vi "Cluster to VArray.vi"(8 "error in (no error)":errorcluster, 10 "Cluster":refnum<class "variant.lvclass">) -> (0 "error out":errorcluster, 2 "VArray":refnum<class "variant.lvclass">)   [LabVIEW 2020, in "variant.lvlib" / "variant.lvclass"]
doc: "Convert a cluster of identical element datatypes into an array."
uses:
  variant.lvclass
  variant.lvclass/variant.ctl
  Type Descriptor/TD.lvclass/TD.ctl
  Bytes/Bytes.lvclass/Bytes.ctl
  Type Descriptor Enumeration.ctl
  Type Descriptor/TD.lvclass
  C:/projects/OpenG-Variant-Data-Library/source/library/Bytes/Bytes.lvclass
  5d20640f-5bd6-45d0-abcc-d5dfbfc7c14e.vi
  Bytes/to_data.vi
  Type Descriptor/get_num_elements.vi/b3898c1b-5169-4cb1-894b-457c92b4a1c3.vi
  Bytes/from_byte_array.vi
  Type Descriptor/get_num_elements.vi/b3898c1b-5169-4cb1-894b-457c92b4a1c3.vi/81433c74-ee36-47cf-a886-10c868675b30.vi
  Type Descriptor/get_num_elements.vi/b3898c1b-5169-4cb1-894b-457c92b4a1c3.vi/d8d9ff34-2c15-4edb-a5ad-7260f11560db.vi
  DataString/DataString.lvclass
  Bytes/Bytes.lvclass
  <userlib>/_OpenG.lib/error/error.llb/openg_error.lvlib
  openg_variant.lvlib
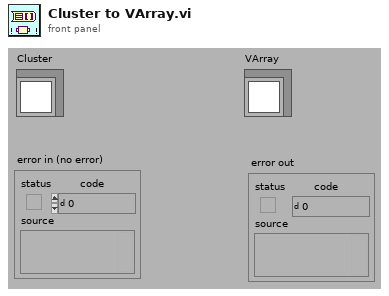
[diagram p1: front panel]
types:
  T1 = typedef "openg_variant.lvlib/Type Descriptor Enumeration.ctl" = enum8{"<Null>", "I8", "I16", "I32", "I64", "U8", "U16", "U32", "U64", "SGL", "DBL", "EXT", "CSG", "CDB", "CXT", "0x0F", "0x10", "0x11", "0x12", "0x13", "0x14", "Enum U8", "Enum U16", "Enum U32", "Enum U64", "SGL PQ", "DBL PQ", "EXT PQ", "CSG PQ", "CDB PQ", "CXT PQ", "0x1F", "0x20", "Boolean", "0x22", "0x23", "0x24", "0x25", "0x26", "0x27", "0x28", "0x29", "0x2A", "0x2B", "0x2C", "0x2D", "0x2E", "0x2F", "String", "0x31", "Path", "Pict", "0x34", "0x35", "0x36", "DAQ", "0x38", "0x39", "0x3A", "0x3B", "0x3C", "0x3D", "0x3E", "0x3F", "Array", "0x41", "0x42", "0x43", "0x44", "0x45", "0x46", "0x47", "0x48", "0x49", "0x4A", "0x4B", "0x4C", "0x4D", "0x4E", "0x4F", "Cluster", "0x51", "0x52", "Variant", "Waveform", "0x55", "0x56", "0x57", "0x58", "0x59", "0x5A", "0x5B", "0x5C", "0x5D", "0x5E", "Fixed Point", "0x60", "0x61", "0x62", "0x63", "0x64", "0x65", "0x66", "0x67", "0x68", "0x69", "0x6A", "0x6B", "0x6C", "0x6D", "0x6E", "0x6F", "Refnum", "0x71", "0x72", "Set Collection", "Map Collection"}
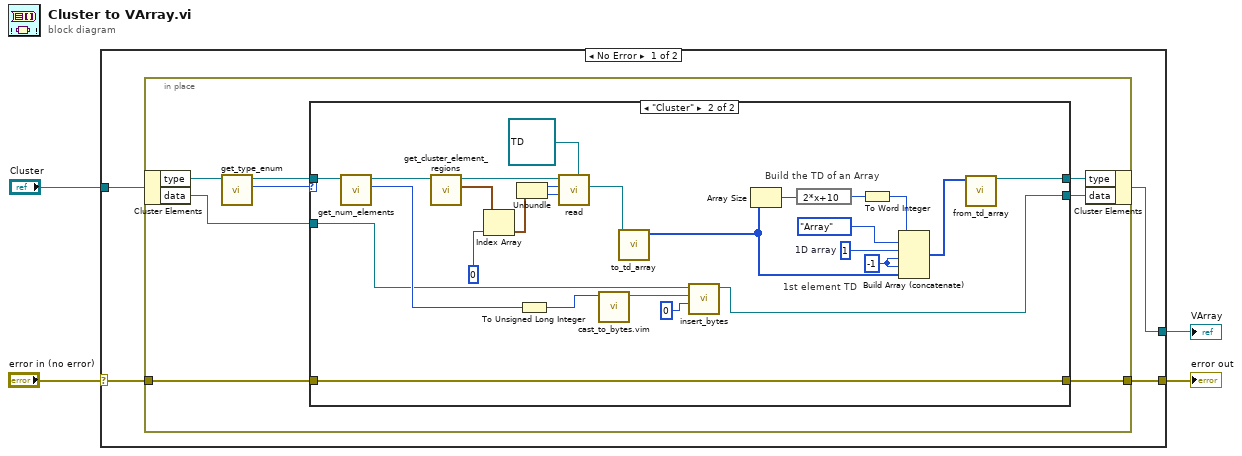
[diagram p0: block diagram]
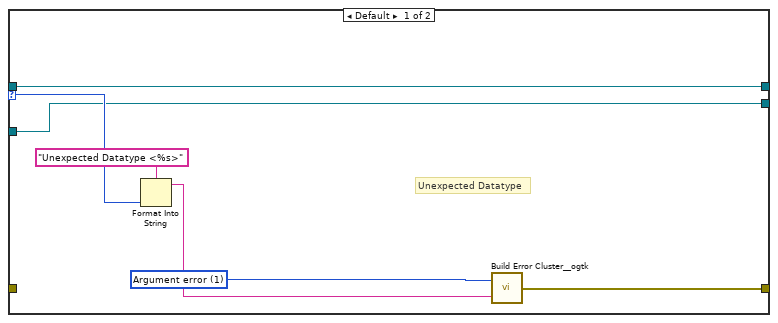
[diagram p2: hidden frame]
diagram:
  n1 = case shown="No Error" "error in (no error)" {
    selector: "error in (no error)" -> [w5 w50]
    tunnel: [w8 w50] -> w4
    tunnel: [w6 _] -> w2
    tunnel: "Cluster" -> [w7 _]
    frame No Error {
      n2 = in-place {
        in-place-border: [w16] -> w8
        in-place-border: w5 -> [w9]
        n3 = in-place-cluster #1(w7) -> ("type"=w15:refnum<class "TD.lvclass">, "data"=w12:refnum<class "DataString.lvclass">)
        n4 = call "get_type_enum.vi"("TypeDescriptor"=w15) -> ("type"=w14:T1, "TypeDescriptor out"=w13:refnum<class "TD.lvclass">)  [unwired: 9 in]
        n5 = case shown="\"Cluster\"" w14 {
          selector: w14 -> [w20 _]
          tunnel: [w23 w24] -> w16
          tunnel: w13 -> [w18 w43]
          tunnel: w12 -> [w17 w31]
          tunnel: [w18 w26] -> w11
          tunnel: [w17 w25] -> w10
          tunnel: w9 -> [_ w24]
          frame Default {
            w22 = 1 items=["No error", "Argument error", "Memory is full", "Out of zone", "End of file", "File already open", "Generic file I/O error", "File not found", "File permission error", "Disk is full", "Duplicate path", "Too many files open", "System feature not enabled", "Resource file not found", "Cannot add resource", "Resource not found", "Image not found", "Image memory error", "Pen does not exist", "Config type invalid", "Config token not found", "Config parse error", "Config memory error", "Bad external code format", "Bad external code offset", "External code not present", "Null window", "Destroy window error", "Null menu", "Print aborted", "Bad print record", "Print driver error", "Windows error during printing", "Memory error during printing", "Print dialog error", "Generic print error", "Invalid device refnum", "Device not found", "Device parameter error", "Device unit error", "Cannot open device", "Device call aborted", "Generic error", "Cancelled by user", "Object ID too low", "Object ID too high", "Object not in heap", "Unknown heap", "Unknown object (invalid DefProc)", "Unknown object (DefProc not in table)", "Message out of range", "Invalid (null) method", "Unknown message", "Manager call not supported", "Bad address", "Network operation in progress", "Network operation timed out", "Connection is busy", "Network attribute not supported", "Network error", "Address in use", "System out of memory", "Connection aborted", "Connection refused", "Not connected", "Already connected", "Connection closed", "Initialization error (interapplication manager)", "Bad occurrence", "Wait on unbound occurrence handler", "Occurrence queue overflow", "Datalog type conflict", "Unused", "Unrecognized type (interapplication manager)", "Memory corrupt", "Failed to make temporary DLL", "Old CIN version", "Drag socket not found", "Failed to load drop-object", "Failed to register OLE object", "Failed to release OLE object", "Format specifier type mismatch", "Unknown format specifier", "Too few format specifiers", "Too many format specifiers", "Scan failed", "Newer CIN version", "Error converting to variant", "Runtime menu error", "Password tampered", "Variant attribute not found", "Incompatible variant data type", "Event data is not available", "Event Store is not present", "Occurrence is not found", "Event Queue is not created", "Event info is not available", "Refnum passed is NULL", "Error retrieving Class GUID", "Error retrieving CoClass GUID", "Error retrieving TypeLib GUID.", "Bad built application magic bytes.", "Specific driver is different from the specific driver associated with the Logical Name.", "There is no session opened to the class driver.", "Max Error", "MAX - Error with config objects", "MAX - Error loading configuration", "MAX - Group not supported"]
            # "Unexpected Datatype"
            n6 = Format Into String(format string="Unexpected Datatype <%s>" ("Format String"), w20) -> (resulting string=w19:string)  [unwired: 2 in, 1 out]
            n7 = call <userlib>:"Build Error Cluster__ogtk.vi"("String to Prepend to source (\"\")"=w19, "code"=w22) -> ("error out"=w23:errorcluster)
          }
          frame "Cluster" {
            w47 = i16 -1 ("Input Element")
            w48 = i16 1  # 1D array
            # "Build the TD of an Array"
            # "1st element TD"
            n8 = call "get_num_elements.vi"("TypeDescriptor"=w43) -> ("num_element"=w42:i32, "TypeDescriptor out"=w41:refnum<class "TD.lvclass">)  [unwired: 9 in]
            n9 = call "get_cluster_element_regions.vi"("TypeDescriptor"=w41) -> ("element_regions"=w40:cluster{i32, i32}[], "TypeDescriptor out"=w39:refnum<class "TD.lvclass">)  [unwired: 8 in, 1 out]
            n10 = Index Array(array=w40, index=0 ("Index")) -> (element=w37:cluster{i32, i32})
            n11 = Unbundle(w37) -> (w35:i32, w36:i32)
            n12 = To Unsigned Long Integer(number=w42) -> (unsigned 32bit integer=w30:u32)
            n13 = call "read.vi"("type to read"=refnum<class "TD.lvclass"> refnum ("TypeDescriptor in"), "length (-1: rest)"=w36, "offset (-1: current position)"=w35, "Bytes in"=w39) -> ("Bytes read"=w34:refnum<class "TD.lvclass">)  [unwired: 6 in, 1 out]
            n14 = call "cast_to_bytes.vim"("anything"=w30) -> ("bytes"=w29:refnum<class "Bytes.lvclass">)  [unwired: 10 in]
            n15 = call "to_td_array.vi"("TypeDescriptor in"=w34) -> ("type string"=w32:i16[])  [unwired: 10 in]
            n16 = call "insert_bytes.vi"("offset (-1: current position)"=0, "bytes to insert"=w29, "Bytes in"=w31) -> ("Bytes out"=w25:refnum<class "DataString.lvclass">)  [unwired: 8 in]
            n17 = Array Size(array=w32) -> (size(s)=w46:i32)
            n18 = expression code="2*x+10"(w46) -> (w45:i32)
            n19 = To Word Integer(number=w45) -> (16bit integer=w44:i16)
            n20 = Build Array (concatenate)(w44, Type_Descriptor_Enumeration."Array" ("Type Descriptor Enumeration"), w48, w47, w47, w32) -> (w27:i16[])
            n21 = call "from_td_array.vi"("type descriptor array"=w27) -> ("TypeDescriptor out"=w26:refnum<class "TD.lvclass">)  [unwired: 9 in, 1 out]
          }
        }
        n22 = in-place-cluster #1("type"=w11, "data"=w10) -> (w6:refnum<class "variant.lvclass">)
      }
    }
    frame Error {
    }
  }
  "error out" <- w4
  "VArray" <- w2
